vi "Utility MODBUS RTU Receive Message.vi"(6 "Receive Message Type (0: By The Number Of Bytes)":u16(ring) items=["By The Number Of Bytes", "Copy Of The Sent Message"], 8 "error in (no error)":errorcluster, 9 "Sent Command (0)":u8, 10 "Length Of Sent MSG (0)":u8, 11 "VISA resource name":refnum<visa-resource-name>) -> (0 "error out":errorcluster, 1 "Read Buffer":u8[](array[numeric]), 3 "VISA resource name out":refnum<visa-resource-name>)   [LabVIEW 2010]
doc: "VI - receive MODBUS RTU frame described by <B>Sent Command</B> control <LengthOfSentMSG> control (set out by MODBUS RTU Send Message.vi) and\nby selection <B>Receive Message Type</B>.\n\nThis VI is without message content decoding.\nSeparate usefull data message\nfrom the rest of the data frame and put it to the <B>read Buffer</B>.\nThe selector decode the frame by type of reading - \n\nAnswers can have 2 types:\n\n1. in answer frame is copy of the frame - is need to initialize on the input - <B>LengthOfSentMSG</B> and <B>Sent Command</B>, for right decoding\n\n2. answer frame consists information about lenth of main message in frame - The frame is divided automaticaly\n\n\nDescribed errors:\nBFFC09F1 - Bad in back protokol in Write Operation. Transmit Error.\nBFFC09F2 - Bad Received Message CRC\nBFFC09F3 - After WRITE: Error Statement, Error CRC\nBFFC09F4 - After WRITE: Register dont exist or is only for reading\nBFFC09F5 - After WRITE: data out of borders"
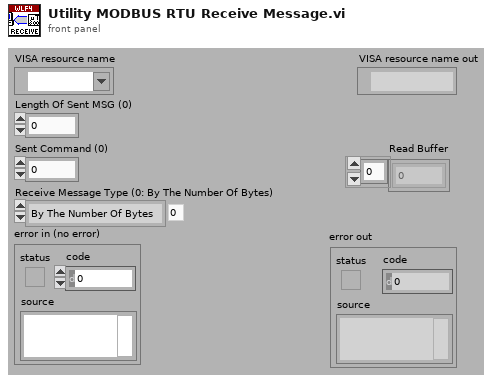
[diagram p1: front panel]
types:
  T1 = cluster{"unsigned byte array[0]":u8, "unsigned byte array[1]":u8}
  T2 = cluster{"status":bool, "code":i32, "VI Name":string}
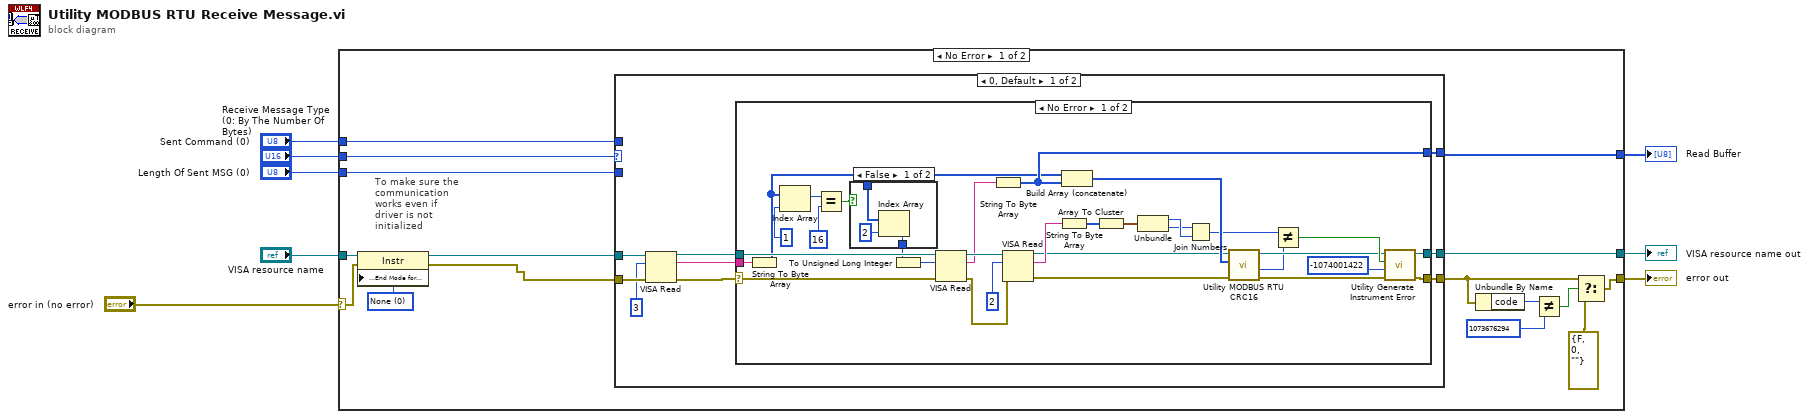
[diagram p0: block diagram]
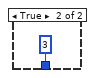
[diagram p2: hidden frame]
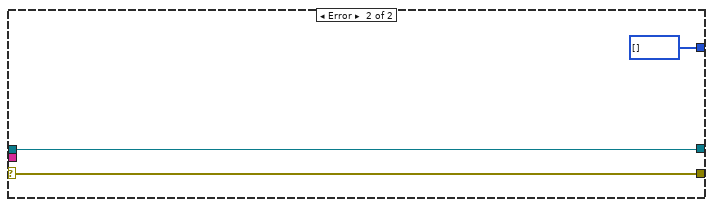
[diagram p3: hidden frame]
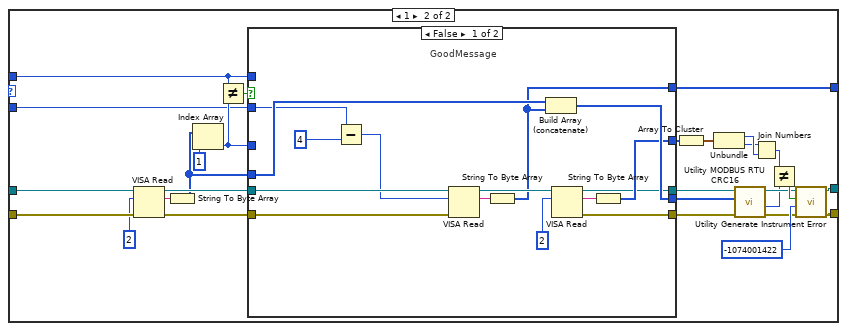
[diagram p4: hidden frame]
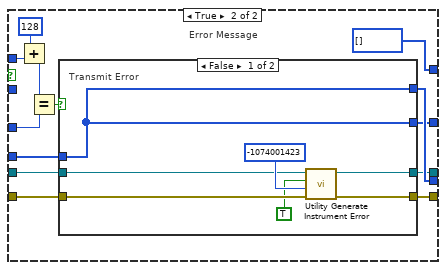
[diagram p5: hidden frame]
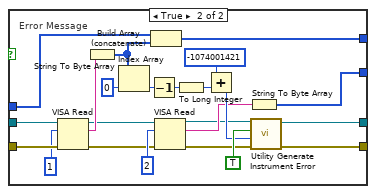
[diagram p6: hidden frame]
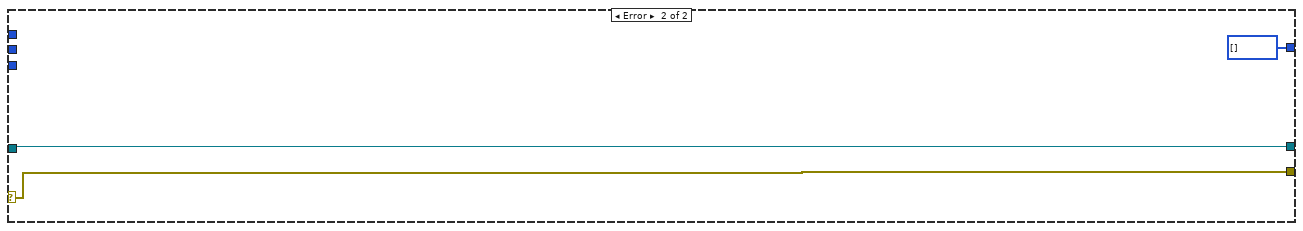
[diagram p7: hidden frame]
diagram:
  n1 = case shown="No Error" "error in (no error)" {
    selector: "error in (no error)" -> [w10 w158]
    tunnel: "Receive Message Type (0: By The Number Of Bytes)" -> [w24 _]
    tunnel: "VISA resource name" -> [w13 w159]
    tunnel: "Length Of Sent MSG (0)" -> [w23 _]
    tunnel: "Sent Command (0)" -> [w22 _]
    tunnel: [w21 u8[] [] ("unsigned byte array")] -> w4
    tunnel: [w15 w159] -> w3
    tunnel: [w14 w158] -> w2
    frame No Error {
      w11 = u16 0 items=["None", "LastBit", "TermChar"] ("Serial Settings:Serial End Mode for Reads")
      # "To make sure the\ncommunication \nworks even if\ndriver is not \ninitialized"
      n2 = property class="Instr"(reference=w13, error in=w10, "Serial Settings:End Mode for Reads"=w11) -> (reference out=w12:refnum<visa-resource-name>, error out=w9:errorcluster)
      n3 = case shown="0, Default" w24 {
        tunnel: [w29 w96] -> w20
        tunnel: w9 -> [w33 w98]
        tunnel: w12 -> [w31 w99]
        tunnel: [w27 w81] -> w15
        tunnel: [w26 w82] -> w21
        tunnel: w23 -> [_ w73]
        tunnel: w22 -> [_ w85]
        frame 0, Default {
          n4 = VISA Read(VISA resource name=w31, byte count=u32 3 ("byte count (0)"), error in (no error)=w33) -> (VISA resource name out=w28:refnum<visa-resource-name>, read buffer=w30:string, error out=w25:errorcluster)  [unwired: 1 out]
          n5 = case shown="No Error" w25 {
            selector: w25 -> [w63 w71]
            tunnel: w30 -> [w64 _]
            tunnel: [w52 w71] -> w29
            tunnel: w28 -> [w62 w70]
            tunnel: [w48 u8[] [] ("unsigned byte array")] -> w26
            tunnel: [w44 w70] -> w27
            frame No Error {
              n6 = String To Byte Array(string=w64) -> (unsigned byte array=w36:u8[])
              n7 = Index Array(array=w36, index=1) -> (element=w38:u8)
              n8 = Equal?(x=w38, y=u8 16 ("x")) -> (x = y?=w37:bool)
              n9 = case shown="False" w37 {
                tunnel: [w66 u8 3] -> w35
                tunnel: w36 -> [w65 _]
                frame False {
                  n10 = Index Array(array=w65, index=2) -> (element=w66:u8)
                }
                frame True {
                }
              }
              n11 = To Unsigned Long Integer(number=w35) -> (unsigned 32bit integer=w41:u32)
              n12 = VISA Read(VISA resource name=w62, byte count=w41, error in (no error)=w63) -> (VISA resource name out=w59:refnum<visa-resource-name>, read buffer=w58:string, error out=w34:errorcluster)  [unwired: 1 out]
              n13 = String To Byte Array(string=w58) -> (unsigned byte array=w48:u8[])
              n14 = VISA Read(VISA resource name=w59, byte count=u32 2 ("byte count (0)"), error in (no error)=w34) -> (VISA resource name out=w46:refnum<visa-resource-name>, read buffer=w61:string, error out=w57:errorcluster)  [unwired: 1 out]
              n15 = String To Byte Array(string=w61) -> (unsigned byte array=w56:u8[])
              n16 = Build Array (concatenate)(w36, w48) -> (w47:u8[])
              n17 = Array To Cluster(array=w56) -> (cluster=w55:T1)
              n18 = Unbundle(w55) -> ("unsigned byte array[0]"=w54:u8, "unsigned byte array[1]"=w53:u8)
              n19 = Join Numbers(hi=w53, lo=w54) -> ((hi.lo)=w43:u16)
              n20 = call "Utility MODBUS RTU CRC16.vi"("error in (no error)"=w57, "Message (empty array)"=w47, "VISA resource name"=w46) -> ("error out"=w50:errorcluster, "CRC"=w42:u16, "VISA resource name out"=w45:refnum<visa-resource-name>)  [unwired: 5 in, 1 out]
              n21 = Not Equal?(x=w43, y=w42) -> (x != y?=w51:bool)
              n22 = call "Utility Generate Instrument Error.vi"("error in (no error)"=w50, "Code (0)"=-1074001422, "Status (F: Off)"=w51, "VISA resource name"=w45) -> ("error out"=w52:errorcluster, "VISA resource name out"=w44:refnum<visa-resource-name>)  [unwired: 6 in]
            }
            frame Error {
            }
          }
        }
        frame 1 {
          n23 = VISA Read(VISA resource name=w99, byte count=u32 2 ("byte count (0)"), error in (no error)=w98) -> (VISA resource name out=w97:refnum<visa-resource-name>, read buffer=w74:string, error out=w72:errorcluster)  [unwired: 1 out]
          n24 = String To Byte Array(string=w74) -> (unsigned byte array=w83:u8[])
          n25 = Index Array(array=w83, index=1) -> (element=w86:u8)
          n26 = Not Equal?(x=w85, y=w86) -> (x != y?=w87:bool)
          n27 = case shown="False" w87 {
            tunnel: w97 -> [w113 w127]
            tunnel: [w105 w118] -> w91
            tunnel: [w110 w120] -> w80
            tunnel: w72 -> [w114 w126]
            tunnel: w86 -> [_ w125]
            tunnel: w85 -> [_ w116]
            tunnel: [w107 w122] -> w84
            tunnel: w83 -> [w112 w121]
            tunnel: [w104 w119] -> w79
            tunnel: [w103 u8[] [] ("unsigned byte array")] -> w82
            tunnel: w73 -> [w102 _]
            frame False {
              # "GoodMessage"
              n28 = Subtract(x=w102, y=u8 4) -> (x-y=w101:u8)
              n29 = VISA Read(VISA resource name=w113, byte count=w101, error in (no error)=w114) -> (VISA resource name out=w109:refnum<visa-resource-name>, read buffer=w111:string)  [unwired: 2 out]
              n30 = String To Byte Array(string=w111) -> (unsigned byte array=w103:u8[])
              n31 = Build Array (concatenate)(w112, w103) -> (w110:u8[])
              n32 = VISA Read(VISA resource name=w109, byte count=u32 2 ("byte count (0)")) -> (VISA resource name out=w104:refnum<visa-resource-name>, read buffer=w106:string, error out=w107:errorcluster)  [unwired: 1 in, 1 out]
              n33 = String To Byte Array(string=w106) -> (unsigned byte array=w105:u8[])
            }
            frame True {
              # "Error Message"
              n34 = Add(x=u8 128 ("y"), y=w116) -> (x+y=w124:u8)
              n35 = Equal?(x=w124, y=w125) -> (x = y?=w123:bool)
              n36 = case shown="False" w123 {
                tunnel: w127 -> [w129 w157]
                tunnel: w126 -> [w133 w156]
                tunnel: [w132 w135] -> w122
                tunnel: w121 -> [w130 w145]
                tunnel: [w130 w144] -> w120
                tunnel: [w128 w136] -> w119
                tunnel: [w130 w141] -> w118
                frame False {
                  # "Transmit Error"
                  n37 = call "Utility Generate Instrument Error.vi"("error in (no error)"=w133, "Code (0)"=-1074001423, "Status (F: Off)"=TRUE ("status"), "VISA resource name"=w129) -> ("error out"=w132:errorcluster, "VISA resource name out"=w128:refnum<visa-resource-name>)  [unwired: 6 in]
                }
                frame True {
                  # "Error Message"
                  n38 = VISA Read(VISA resource name=w157, byte count=u32 1 ("byte count (0)"), error in (no error)=w156) -> (VISA resource name out=w140:refnum<visa-resource-name>, read buffer=w153:string, error out=w139:errorcluster)  [unwired: 1 out]
                  n39 = String To Byte Array(string=w153) -> (unsigned byte array=w152:u8[])
                  n40 = Index Array(array=w152, index=0) -> (element=w150:u8)
                  n41 = Decrement(x=w150) -> (x-1=w147:u8)
                  n42 = Build Array (concatenate)(w145, w152) -> (w144:u8[])
                  n43 = VISA Read(VISA resource name=w140, byte count=u32 2 ("byte count (0)"), error in (no error)=w139) -> (VISA resource name out=w137:refnum<visa-resource-name>, read buffer=w142:string, error out=w138:errorcluster)  [unwired: 1 out]
                  n44 = To Long Integer(number=w147) -> (32bit integer=w146:i32)
                  n45 = Add(x=-1074001421, y=w146) -> (x+y=w148:i32)
                  n46 = String To Byte Array(string=w142) -> (unsigned byte array=w141:u8[])
                  n47 = call "Utility Generate Instrument Error.vi"("error in (no error)"=w138, "Code (0)"=w148, "Status (F: Off)"=TRUE ("status"), "VISA resource name"=w137) -> ("error out"=w135:errorcluster, "VISA resource name out"=w136:refnum<visa-resource-name>)  [unwired: 6 in]
                }
              }
            }
          }
          n48 = Array To Cluster(array=w91) -> (cluster=w94:T1)
          n49 = Unbundle(w94) -> ("unsigned byte array[0]"=w93:u8, "unsigned byte array[1]"=w92:u8)
          n50 = call "Utility MODBUS RTU CRC16.vi"("error in (no error)"=w84, "Message (empty array)"=w80, "VISA resource name"=w79) -> ("error out"=w89:errorcluster, "CRC"=w77:u16, "VISA resource name out"=w78:refnum<visa-resource-name>)  [unwired: 5 in, 1 out]
          n51 = Join Numbers(hi=w92, lo=w93) -> ((hi.lo)=w76:u16)
          n52 = Not Equal?(x=w76, y=w77) -> (x != y?=w90:bool)
          n53 = call "Utility Generate Instrument Error.vi"("error in (no error)"=w89, "Code (0)"=-1074001422, "Status (F: Off)"=w90, "VISA resource name"=w78) -> ("error out"=w96:errorcluster, "VISA resource name out"=w81:refnum<visa-resource-name>)  [unwired: 6 in]
        }
      }
      n54 = Unbundle By Name(w20) -> ("code"=w19:i32)
      n55 = Not Equal?(x=w19, y=1073676294) -> (x != y?=w17:bool)
      n56 = Select(t=w20, s=w17, f=cluster{bool, i32, "VI Name":string} {FALSE, 0, "VI Name"=""}) -> (s? t:f=w14:T2)
    }
    frame Error {
    }
  }
  "error out" <- w2
  "VISA resource name out" <- w3
  "Read Buffer" <- w4
